vi "Database Insert.vi"() -> ()   [LabVIEW 2018]
doc: "This example allows you to perform several tasks on the specified table in a database named LabVIEW.mdb located in the LabVIEW examples>>database directory.\n\nThis VI is running when you open it. Select one of the tabs and enter the appropriate data. Press the Go button to complete the displayed tab option.\n\nAutomatic - This option inserts a new record into the specified table. The record is specified by a cluster containing the correct number of elements and of the data types defined by the specified table. \n\nSQL Query - This option performs the specified SQL query.\n\nParameterized SQL Query - This option performs the specified SQL query as a parameterized SQL Query. This method is faster and more efficient than directly executing an SQL query because it sets up all the parameters prior to doing the command."
uses:
  <vilib>/addons/database/Auxilliary.llb/DB Tools Parameter Info.ctl
  <vilib>/addons/database/Auxilliary.llb/DB Tools DataTypes.ctl
  <vilib>/addons/database/Auxilliary.llb/DB Tools Parameter Dir.ctl
  <vilib>/addons/database/Connection.llb/DB Tools Open Connec (Path).vi
  <vilib>/addons/database/Connection.llb/Conn Execute.vi
  <vilib>/addons/database/Recordset.llb/Rec Destroy - Connection.vi
  <vilib>/addons/database/Command.llb/Cmd Set Parameter Value (C).vi
  <vilib>/addons/database/Command.llb/Cmd Execute.vi
  <vilib>/addons/database/Recordset.llb/Rec Destroy - Command.vi
  <vilib>/addons/database/Command.llb/Cmd Delete.vi
  <vilib>/addons/database/NI_Database_API.lvlib
panel:
  in  "Data":T1={"query type"="automatic", "device name"="mydevice", "number of samples"=1024}
  in  "Parameterized SQL query":string="insert into inserttable (querytype, device, numsamples) values ('parameterized sql query', ?, ?) "
  in  "parameters":T2[](array[typedef])=[{"parameter name"="", "type"=enum."String", "direction"=enum."Input", "value"=variant}, {"parameter name"="", "type"=enum."Long (I32)", "direction"=enum."Input", "value"=variant}]
  in  "device name":string="mydevice"
  in  "number of samples":i32=2048
  in  "SQL query":string="insert into inserttable (querytype, device, numsamples) values ('sql query', 'mydevice', 1872) "
  # "Overview: Demonstrates how to insert records into databases, and perform SQL queries.\nRequirements: Database Connectivity Toolkit\nInstructions:\nRun the VI."
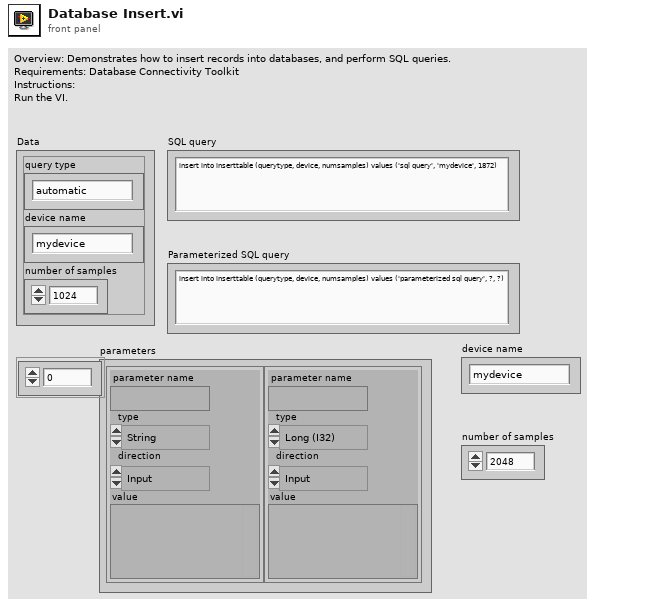
[diagram p1: front panel]
types:
  T1 = cluster{"query type":string, "device name":string, "number of samples":i32}
  T2 = typedef "NI_Database_API.lvlib/DB Tools Parameter Info.ctl" = cluster{"parameter name":string, "type":T3, "direction":T4, "value":variant}
  T3 = typedef "NI_Database_API.lvlib/DB Tools DataTypes.ctl" = enum16{"String", "Long (I32)", "Single (SGL)", "Double (DBL)", "Date/Time", "Binary"}
  T4 = typedef "NI_Database_API.lvlib/DB Tools Parameter Dir.ctl" = enum32{"Input", "Output", "Input/Output", "Return Value"}
  T5 = typedef "NI_Database_API.lvlib/Conn ObjectReference.ctl" = refnum<k1>
  T6 = typedef "NI_Database_API.lvlib/Rec ObjectReference.ctl" = refnum<k1>
  T7 = typedef "NI_Database_API.lvlib/Cmd ObjectReference.ctl" = refnum<k1>
  T8 = typedef "NI_Database_API.lvlib/Cmd-Rec Object Reference.ctl" = refnum<k1>
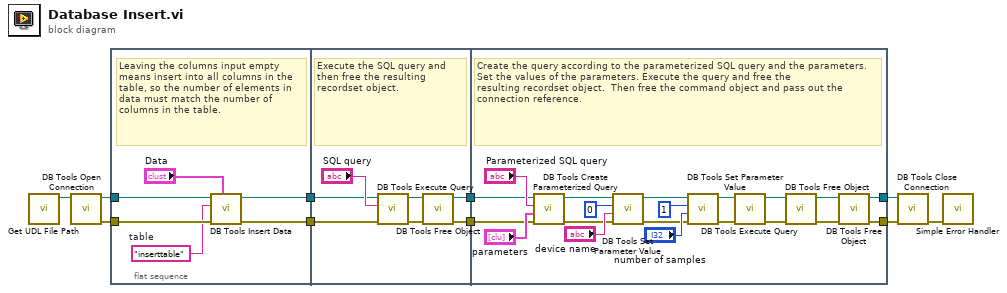
[diagram p0: block diagram]
diagram:
  n1 = call "Get UDL File Path.vi"() -> ("UDL file path"=w8:path)  [unwired: 11 in]
  n2 = call-poly <vilib>:"DB Tools Open Connection.vi"("connection information"=w8) -> ("error out"=w5:errorcluster, "connection reference"=w6:T5)  [unwired: 7 in]
  n3 = flat-sequence {
    tunnel: w6 -> [w14]
    tunnel: w5 -> [w13]
    tunnel: [w16] -> w4
    tunnel: [w15] -> w3
    tunnel: w4 -> [w20]
    tunnel: w3 -> [w19]
    tunnel: [w17] -> w2
    tunnel: [w18] -> w1
    tunnel: [w27] -> w7
    tunnel: [w24] -> w10
    tunnel: w2 -> [w29]
    tunnel: w1 -> [w30]
    frame #0 {
      w12 = "inserttable"  # table
      # "Leaving the columns input empty means insert into all columns in the table, so the number of elements in\ndata must match the number of columns in the table."
      n4 = call <vilib>:"DB Tools Insert Data.vi"("data"="Data", "error in (no error)"=w13, "table"=w12, "connection reference"=w14) -> ("error out"=w16:errorcluster, "connection reference out"=w15:T5)  [unwired: 6 in]
    }
    frame #1 {
      # "Execute the SQL query and then free the resulting recordset object."
      n5 = call-poly <vilib>:"DB Tools Execute Query.vi"("error in (no error)"=w20, "SQL query"="SQL query", "connection reference"=w19) -> ("error out"=w21:errorcluster, "recordset reference"=w22:T6)  [unwired: 5 in]
      n6 = call-poly <vilib>:"DB Tools Free Object.vi"("error in (no error)"=w21, "recordset reference"=w22) -> ("error out"=w17:errorcluster, "connection reference"=w18:T5)  [unwired: 8 in]
    }
    frame #2 {
      # "Create the query according to the parameterized SQL query and the parameters. Set the values of the parameters. Execute the query and free the \nresulting recordset object.  Then free the command object and pass out the connection reference."
      n7 = call <vilib>:"DB Tools Create Parameterized Query.vi"("error in (no error)"=w29, "parameters"="parameters", "SQL query"="Parameterized SQL query", "connection reference"=w30) -> ("error out"=w32:errorcluster, "command reference"=w38:T7)  [unwired: 3 in, 1 out]
      n8 = call-poly <vilib>:"DB Tools Set Parameter Value.vi"("error in (no error)"=w32, "value"="device name", "parameter index"=0, "command reference"=w38) -> ("error out"=w34:errorcluster, "command reference out"=w33:T7)  [unwired: 4 in]
      n9 = call-poly <vilib>:"DB Tools Set Parameter Value.vi"("error in (no error)"=w34, "value"="number of samples", "parameter index"=1, "command reference"=w33) -> ("error out"=w41:errorcluster, "command reference out"=w40:T7)  [unwired: 4 in]
      n10 = call-poly <vilib>:"DB Tools Execute Query.vi"("error in (no error)"=w41, "command reference"=w40) -> ("error out"=w39:errorcluster, "command-recordset reference"=w42:T8)  [unwired: 6 in]
      n11 = call-poly <vilib>:"DB Tools Free Object.vi"("error in (no error)"=w39, "command-recordset reference"=w42) -> ("error out"=w28:errorcluster, "command reference"=w43:T7)  [unwired: 8 in]
      n12 = call-poly <vilib>:"DB Tools Free Object.vi"("error in (no error)"=w28, "command reference"=w43) -> ("error out"=w24:errorcluster, "connection reference"=w27:T5)  [unwired: 8 in]
    }
  }
  n13 = call <vilib>:"DB Tools Close Connection.vi"("error in (no error)"=w10, "connection reference"=w7) -> ("error out"=w9:errorcluster)  [unwired: 5 in]
  n14 = call <vilib>:"Simple Error Handler.vi"("error in (no error)"=w9) -> ()  [unwired: 4 in, 5 out]
